vi "AuMT8852B Tester Modulation Index.vi"(5 "Index (0.35)":dbl=0.35 format="%.2f", 7 "Set/Get (Set)":enum16{"Set", "Get"}(ring), 8 "error in (no error)":errorcluster, 11 "VISA session":refnum<visa-resource-name>) -> (0 "error out":errorcluster, 2 "error code":i32, 3 "VISA session out":refnum<visa-resource-name>, 4 "Index out":dbl=0.35 format="%.2f")   [LabVIEW 2017]
doc: "Anritsu MT8852B Bluetooth Tester\n\nSets or queries the modulation index of the Bluetooth tester.\n\nINPUTS\nSet/Get - whether the value is being sent to or retrieved from the instrument.\nIndex - information to send to the instrument.\n\nOUTPUTS\nIndex out - current value in the instrument."
uses:
  <instrlib>/aumt8852B/General/Utilities/MT8850 Attribute ID.ctl
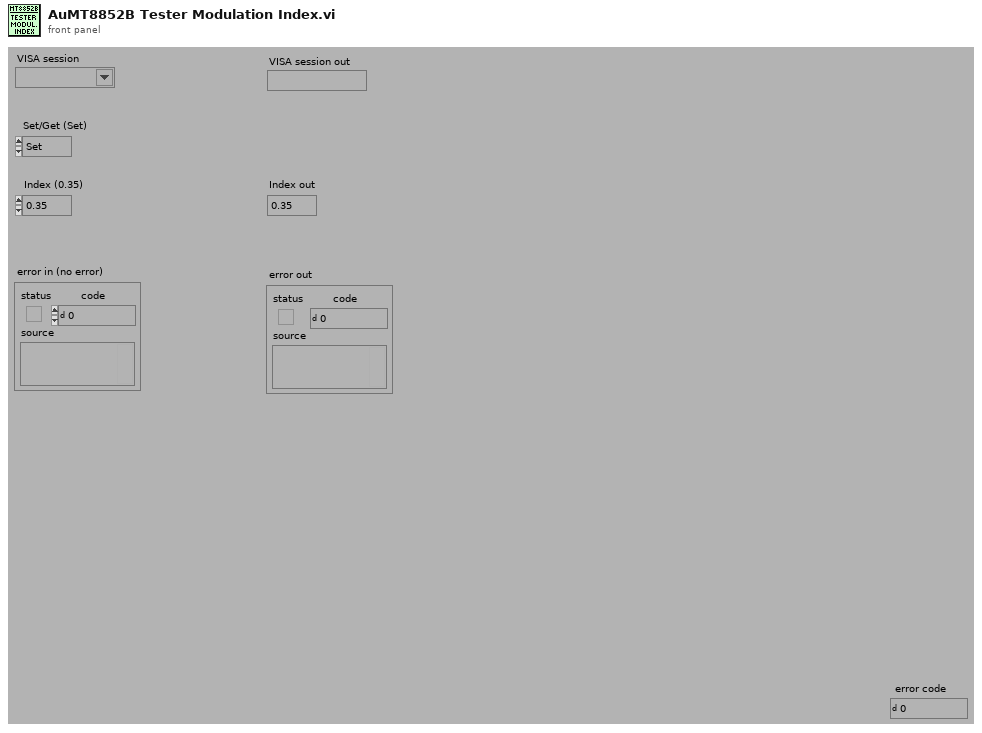
[diagram p1: front panel]
types:
  T1 = typedef "MT8850 Attribute ID.ctl" = enum16{"Operation mode", "Selected script", "EUT address source", "EUT Address", "EUT HCI RS232 Baud Rate", "Tester GPIB Address", "Tester RS232 Baud Rate", "Tester Bluetooth Address", "Tester Contrast", "Tester Key Click On", "Tester Modulation Index", "Tester Poll-Null Mode", "Tester Power Range", "Tester RS232 Mode", "Beep on Illegal Entry", "Display User Text", "User Text", "Calibration TX Modulation DAC", "Calibration RX Channel", "Calibration TX Channel", "Calibration TX Power", "Calibration Use TX Table", "Inquiry Request User-friendly Name", "Inquiry Number of Responses", "Inquiry Timeout", "Script Frequency Display", "Script Loop Count", "Script Loop Continuously", "Script Loop Stop on Fail", "Link timeout", "Page timeout", "Filter bandwidth", "SCO air code", "SCO bit position", "SCO input code", "SCO input data", "SCO input sample size", "SCO loopback mode", "SCO packet type", "SCO tone generator", "Tester page scan repetition mode", "Tester follow test mode", "Tester authentication state", "Tester authentication pin code", "Tester authentication pin length"}
  T2 = typedef "Attribute Status.ctl" = enum16{"No I/O needed", "I/O needed"}
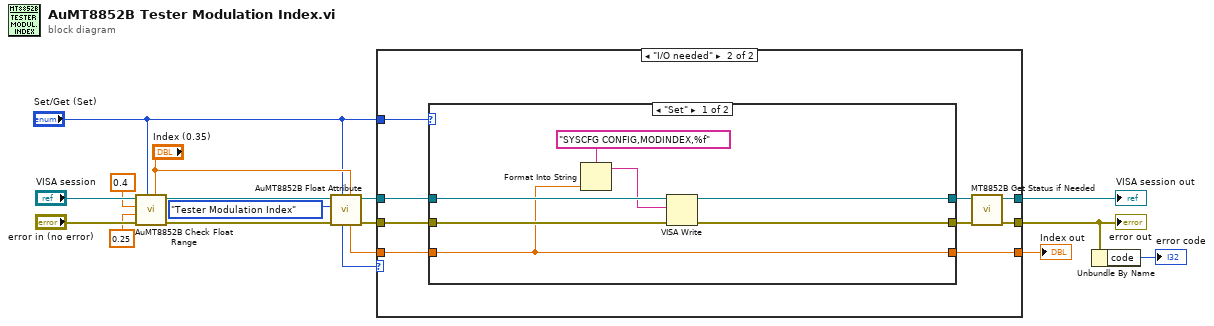
[diagram p0: block diagram]
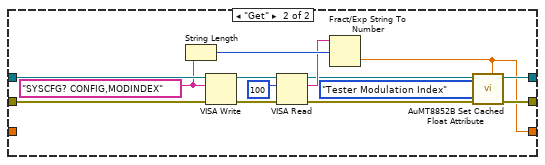
[diagram p3: hidden frame]
diagram:
  n1 = call <instrlib>:"AuMT8852B Check Float Range.vi"("Value (0)"="Index (0.35)", "Set/Get (Set)"="Set/Get (Set)", "error in (no error)"="error in (no error)", "Lower limit (-1)"=0.25, "Upper limit (1)"=0.4, "VISA session"="VISA session") -> ("error out"=w8:errorcluster, "VISA session out"=w9:refnum<visa-resource-name>)  [unwired: 4 in]
  n2 = call <instrlib>:"AuMT8852B Float Attribute.vi"("Value (0.00)"="Index (0.35)", "Set/Get (Set)"="Set/Get (Set)", "error in (no error)"=w8, "Attribute ID"=MT8850_Attribute_ID."Tester Modulation Index", "VISA session"=w9) -> ("error out"=w13:errorcluster, "VISA session out"=w14:refnum<visa-resource-name>, "Value out"=w16:dbl, "Status"=w12:T2)  [unwired: 3 in]
  n3 = case shown="\"I/O needed\"" w12 {
    tunnel: w16 -> [w18 w27]
    tunnel: [w19 w23] -> w3
    tunnel: [w20 w24] -> w15
    tunnel: w14 -> [w20 w29]
    tunnel: w13 -> [w19 w28]
    tunnel: "Set/Get (Set)" -> [_ w22]
    tunnel: [w18 w21] -> w1
    frame "No I/O needed", Default {
    }
    frame "I/O needed" {
      n4 = case shown="\"Set\"" w22 {
        tunnel: w29 -> [w36 w49]
        tunnel: w28 -> [w35 w50]
        tunnel: w27 -> [w30 _]
        tunnel: [w34 w41] -> w26
        tunnel: [w33 w42] -> w25
        tunnel: [w30 w38] -> w21
        frame "Set" {
          n5 = Format Into String(format string="SYSCFG CONFIG,MODINDEX,%f" ("Format String"), w30) -> (resulting string=w31:string)  [unwired: 2 in, 1 out]
          n6 = VISA Write(VISA resource name=w36, write buffer=w31, error in (no error)=w35) -> (VISA resource name out=w34:refnum<visa-resource-name>, error out=w33:errorcluster)  [unwired: 1 out]
        }
        frame "Get" {
          w45 = "SYSCFG? CONFIG,MODINDEX" ("write buffer (\"\")")
          n7 = String Length(string=w45) -> (length=w44:i32)
          n8 = VISA Write(VISA resource name=w49, write buffer=w45, error in (no error)=w50) -> (VISA resource name out=w47:refnum<visa-resource-name>, error out=w48:errorcluster)  [unwired: 1 out]
          n9 = VISA Read(VISA resource name=w47, byte count=u32 100 ("byte count (0)"), error in (no error)=w48) -> (VISA resource name out=w40:refnum<visa-resource-name>, read buffer=w43:string, error out=w39:errorcluster)  [unwired: 1 out]
          n10 = Fract/Exp String To Number(string=w43, offset=w44) -> (number=w38:dbl)  [unwired: 2 in, 1 out]
          n11 = call <instrlib>:"AuMT8852B Set Cached Float Attribute.vi"("Value (0)"=w38, "error in (no error)"=w39, "Attribute ID"=MT8850_Attribute_ID."Tester Modulation Index", "VISA session"=w40) -> ("error out"=w42:errorcluster, "VISA session out"=w41:refnum<visa-resource-name>)  [unwired: 6 in]
        }
      }
      n12 = call <instrlib>:"MT8852B Get Status if Needed.vi"("error in (no error)"=w25, "VISA session"=w26) -> ("error out"=w23:errorcluster, "VISA session out"=w24:refnum<visa-resource-name>)  [unwired: 8 in]
    }
  }
  "error out" <- w3
  "VISA session out" <- w15
  "Index out" <- w1
  n13 = Unbundle By Name(w3) -> ("code"=→"error code":i32)
